vi "GEA3 HEWH Standard ERDs.vi"(8 "Error In":errorcluster, 10 "ERD Data Input":T1[](array[typedef]) {"ERD Number" format="%.0x"}, 11 "ERD Data  in":T2) -> (0 "Error Out":errorcluster, 2 "ERD Data Output":T1[](array[typedef]) {"ERD Number" format="%.0x"}, 3 "ERD Data  out":T2, 5 "Standard Data":string[][](array[string]))   [LabVIEW 2020]
uses:
  type defs/ERD Read Data Out.ctl
  Type Definitions/GEA3 HEWH ERD Data.ctl
  Type Definitions/GEA3 HEWH Mixing Valve.ctl
  library/GEA2_Toolkit.lvlib
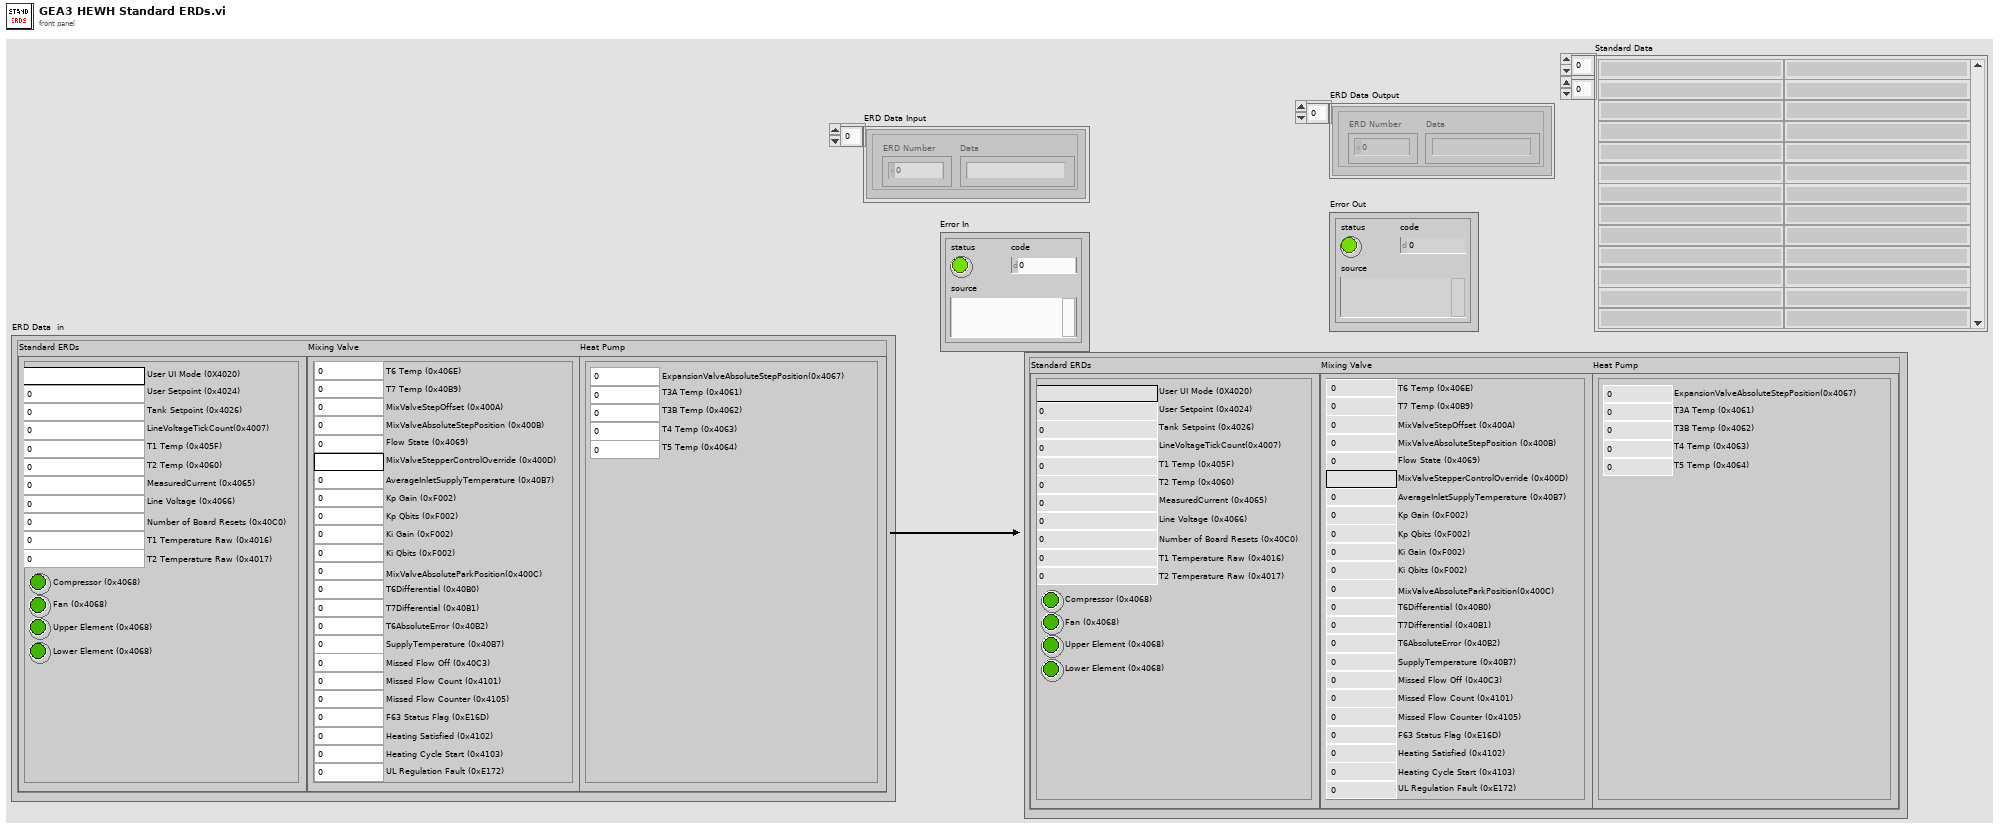
[diagram p1: front panel]
types:
  T1 = typedef "GEA2_Toolkit.lvlib/ERD Read Data Out.ctl" = cluster{"ERD Number":u16, "Data":string}
  T2 = typedef "GEA3 HEWH ERD Data.ctl" = cluster{"Mixing Valve":T3, "Standard ERDs":cluster{"User UI Mode (0X4020)":string, "User Setpoint (0x4024)":u16, "Compressor (0x4068)":bool, "Lower Element (0x4068)":bool, "Upper Element (0x4068)":bool, "Fan (0x4068)":bool, "T1 Temp (0x405F)":dbl, "T2 Temp (0x4060)":dbl, "Line Voltage (0x4066)":dbl, "MeasuredCurrent (0x4065)":dbl, "LineVoltageTickCount(0x4007)":u16, "Number of Board Resets (0x40C0)":u16, "T1 Temperature Raw (0x4016)":u16, "T2 Temperature Raw (0x4017)":u16, "Tank Setpoint (0x4026)":u16}, "Heat Pump":cluster{"ExpansionValveAbsoluteStepPosition(0x4067)":i16, "T3A Temp (0x4061)":dbl, "T3B Temp (0x4062)":dbl, "T4 Temp (0x4063)":dbl, "T5 Temp (0x4064)":dbl}}
  T3 = typedef "GEA3 HEWH Mixing Valve.ctl" = cluster{"T7 Temp (0x40B9)":dbl, "MixValveStepOffset (0x400A)":i16, "MixValveAbsoluteStepPosition (0x400B)":i16, "Flow State (0x4069)":u8, "MixValveStepperControlOverride (0x400D)":string, "AverageInletSupplyTemperature (0x40B7)":dbl, "T6 Temp (0x406E)":dbl, "Kp Gain (0xF002)":u16, "Kp Qbits (0xF002)":u16, "Ki Gain (0xF002)":u16, "Ki Qbits (0xF002)":u16, "MixValveAbsoluteParkPosition(0x400C)":i16, "T7Differential (0x40B1)":dbl, "T6Differential (0x40B0)":dbl, "SupplyTemperature (0x40B7)":dbl, "Missed Flow Off (0x40C3)":u8, "T6AbsoluteError (0x40B2)":dbl, "Missed Flow Count (0x4101)":u16, "Missed Flow Counter (0x4105)":u16, "F63 Status Flag (0xE16D)":u16, "Heating Satisfied (0x4102)":u16, "Heating Cycle Start (0x4103)":u16, "UL Regulation Fault (0xE172)":u8}
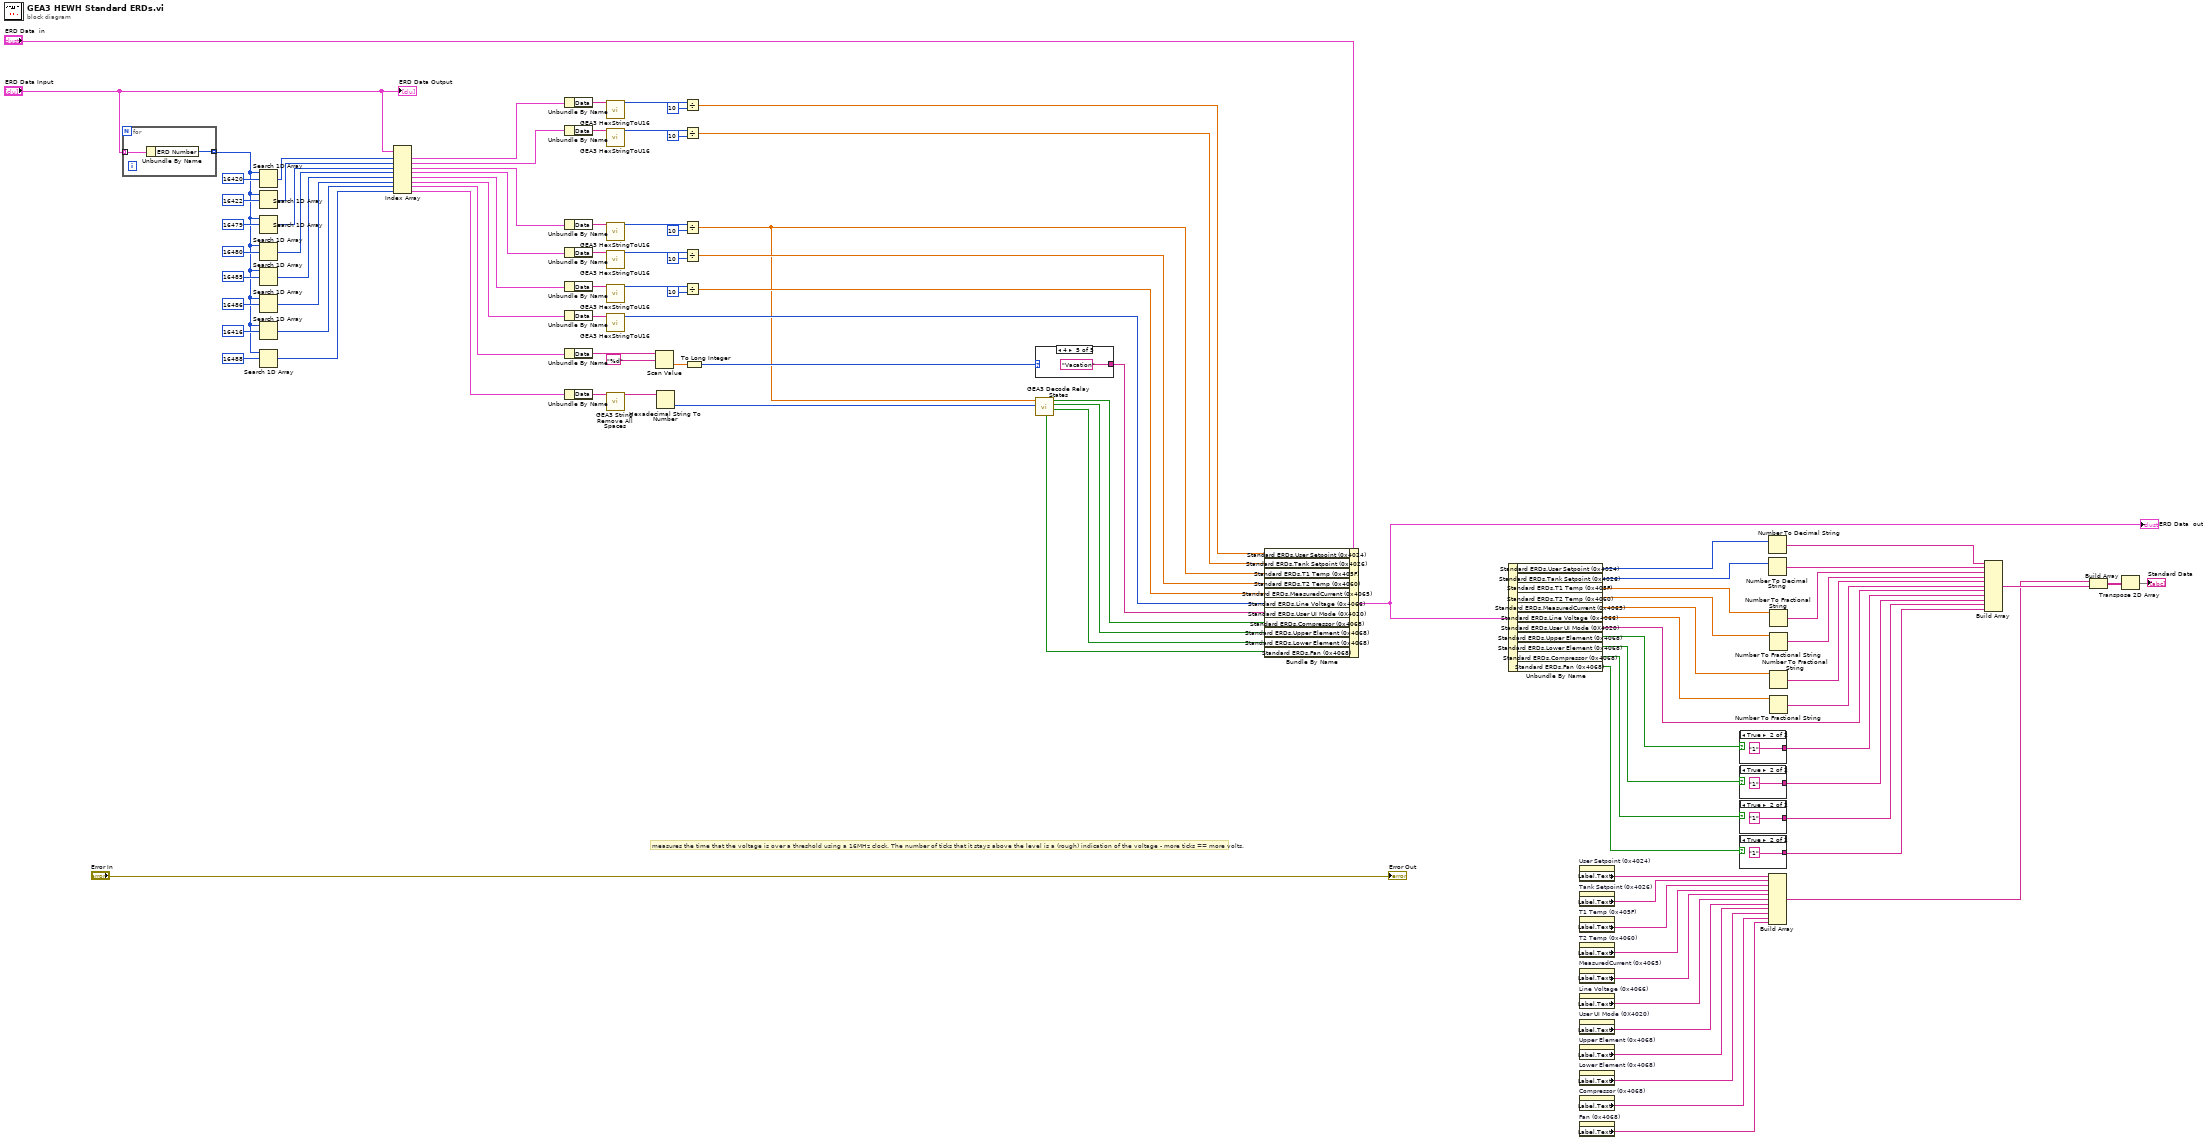
[diagram p0: block diagram]
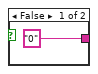
[diagram p2: hidden frame]
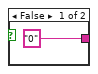
[diagram p3: hidden frame]
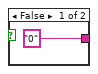
[diagram p4: hidden frame]
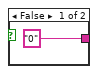
[diagram p5: hidden frame]
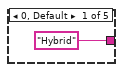
[diagram p6: hidden frame]
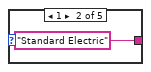
[diagram p7: hidden frame]
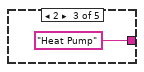
[diagram p8: hidden frame]
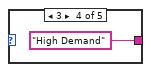
[diagram p9: hidden frame]
diagram:
  # "measures the time that the voltage is over a threshold using a 16MHz clock. The number of ticks that it stays above the level is a (rough) indication of the voltage - more ticks == more volts."
  n1 = for {
    tunnel: "ERD Data Input" -> [w101] mode=indexing
    tunnel: [w100] -> w23 mode=indexing
    n2 = Unbundle By Name(w101) -> ("ERD Number"=w100:u16)
  }
  n3 = Search 1D Array(1D array=w23, element=u16 16420 ("ERD Number")) -> (index of element=w43:i32)  [unwired: 1 in]
  n4 = Search 1D Array(1D array=w23, element=u16 16422 ("ERD Number")) -> (index of element=w31:i32)  [unwired: 1 in]
  n5 = Search 1D Array(1D array=w23, element=u16 16479 ("ERD Number")) -> (index of element=w22:i32)  [unwired: 1 in]
  n6 = Search 1D Array(1D array=w23, element=u16 16480 ("ERD Number")) -> (index of element=w21:i32)  [unwired: 1 in]
  n7 = Search 1D Array(1D array=w23, element=u16 16485 ("ERD Number")) -> (index of element=w20:i32)  [unwired: 1 in]
  n8 = Search 1D Array(1D array=w23, element=u16 16486 ("ERD Number")) -> (index of element=w19:i32)  [unwired: 1 in]
  n9 = Search 1D Array(1D array=w23, element=u16 16416 ("ERD Number")) -> (index of element=w18:i32)  [unwired: 1 in]
  n10 = Search 1D Array(1D array=w23, element=u16 16488 ("ERD Number")) -> (index of element=w17:i32)  [unwired: 1 in]
  n11 = Index Array(array="ERD Data Input", index #1=w43, index #2=w31, index #3=w22, index #4=w21, index #5=w20, index #6=w19, index #7=w18, index #8=w17) -> (element #1=w42:T1, element #2=w27:T1, element #3=w16:T1, element #4=w15:T1, element #5=w14:T1, element #6=w13:T1, element #7=w12:T1, element #8=w11:T1)
  n12 = Unbundle By Name(w42) -> ("Data"=w79:string)
  n13 = Unbundle By Name(w27) -> ("Data"=w28:string)
  n14 = Unbundle By Name(w16) -> ("Data"=w75:string)
  n15 = Unbundle By Name(w15) -> ("Data"=w81:string)
  n16 = Unbundle By Name(w14) -> ("Data"=w86:string)
  n17 = Unbundle By Name(w13) -> ("Data"=w88:string)
  n18 = Unbundle By Name(w12) -> ("Data"=w90:string)
  n19 = Unbundle By Name(w11) -> ("Data"=w94:string)
  n20 = call "GEA3 HexStringToU16.vi"("Input String"=w79) -> ("Number Out"=w77:u16)  [unwired: 14 in]
  n21 = call "GEA3 HexStringToU16.vi"("Input String"=w28) -> ("Number Out"=w30:u16)  [unwired: 14 in]
  n22 = call "GEA3 HexStringToU16.vi"("Input String"=w75) -> ("Number Out"=w73:u16)  [unwired: 14 in]
  n23 = call "GEA3 HexStringToU16.vi"("Input String"=w81) -> ("Number Out"=w83:u16)  [unwired: 14 in]
  n24 = call "GEA3 HexStringToU16.vi"("Input String"=w86) -> ("Number Out"=w85:u16)  [unwired: 14 in]
  n25 = call "GEA3 HexStringToU16.vi"("Input String"=w88) -> ("Number Out"=w89:u16)  [unwired: 14 in]
  n26 = call "GEA3 String Remove All Spaces.vi"("Input String"=w94) -> ("Spaces Removed"=w93:string)  [unwired: 13 in, 1 out]
  n27 = Scan Value(string=w90, format string="%d") -> (value=w95:dbl)  [unwired: 1 in, 1 out]
  n28 = Hexadecimal String To Number(string=w93) -> (number=w92:u32)  [unwired: 2 in, 1 out]
  n29 = Divide(x=w77, y=u16 10) -> (x/y=w80:dbl)
  n30 = Divide(x=w30, y=u16 10) -> (x/y=w26:dbl)
  n31 = Divide(x=w73, y=u16 10) -> (x/y=w64:dbl)
  n32 = Divide(x=w83, y=u16 10) -> (x/y=w76:dbl)
  n33 = Divide(x=w85, y=u16 10) -> (x/y=w87:dbl)
  n34 = To Long Integer(number=w95) -> (32bit integer=w96:i32)
  n35 = case shown="4" w96 {
    tunnel: ["Hybrid" "Standard Electric" "Heat Pump" "High Demand" "Vacation"] -> w97
    frame 0, Default {
    }
    frame 1 {
    }
    frame 2 {
    }
    frame 3 {
    }
    frame 4 {
    }
  }
  n36 = call "GEA3 Decode Relay States.vi"("ERD Relay Value"=w92, "T1 Temp"=w64) -> ("Lower Element (0x4033)"=w39:bool, "Upper Element (0x4033)"=w38:bool, "Compressor (0x4033)"=w40:bool, "Fan (0x4033)"=w37:bool)  [unwired: 6 in]
  n37 = Bundle By Name(cluster="ERD Data  in", "Standard ERDs.User Setpoint (0x4024)"=w80, "Standard ERDs.Tank Setpoint (0x4026)"=w26, "Standard ERDs.T1 Temp (0x405F)"=w64, "Standard ERDs.T2 Temp (0x4060)"=w76, "Standard ERDs.MeasuredCurrent (0x4065)"=w87, "Standard ERDs.Line Voltage (0x4066)"=w89, "Standard ERDs.User UI Mode (0X4020)"=w97, "Standard ERDs.Compressor (0x4068)"=w40, "Standard ERDs.Upper Element (0x4068)"=w38, "Standard ERDs.Lower Element (0x4068)"=w39, "Standard ERDs.Fan (0x4068)"=w37) -> (w63:T2)
  "ERD Data  out" <- w63
  n38 = Unbundle By Name(w63) -> ("Standard ERDs.User Setpoint (0x4024)"=w62:u16, "Standard ERDs.Tank Setpoint (0x4026)"=w25:u16, "Standard ERDs.T1 Temp (0x405F)"=w61:dbl, "Standard ERDs.T2 Temp (0x4060)"=w60:dbl, "Standard ERDs.MeasuredCurrent (0x4065)"=w59:dbl, "Standard ERDs.Line Voltage (0x4066)"=w58:dbl, "Standard ERDs.User UI Mode (0X4020)"=w52:string, "Standard ERDs.Upper Element (0x4068)"=w51:bool, "Standard ERDs.Lower Element (0x4068)"=w49:bool, "Standard ERDs.Compressor (0x4068)"=w36:bool, "Standard ERDs.Fan (0x4068)"=w35:bool)
  n39 = property on="User Setpoint (0x4024)" class="DigNum (strict)"() -> ("Label.Text"=w41:string)  [unwired: 2 in, 2 out]
  n40 = property on="Tank Setpoint (0x4026)" class="DigNum (strict)"() -> ("Label.Text"=w10:string)  [unwired: 2 in, 2 out]
  n41 = property on="T1 Temp (0x405F)" class="DigNum (strict)"() -> ("Label.Text"=w9:string)  [unwired: 2 in, 2 out]
  n42 = property on="T2 Temp (0x4060)" class="DigNum (strict)"() -> ("Label.Text"=w8:string)  [unwired: 2 in, 2 out]
  n43 = property on="MeasuredCurrent (0x4065)" class="DigNum (strict)"() -> ("Label.Text"=w7:string)  [unwired: 2 in, 2 out]
  n44 = property on="Line Voltage (0x4066)" class="DigNum (strict)"() -> ("Label.Text"=w6:string)  [unwired: 2 in, 2 out]
  n45 = property on="User UI Mode (0X4020)" class="Str"() -> ("Label.Text"=w5:string)  [unwired: 2 in, 2 out]
  n46 = property on="Upper Element (0x4068)" class="Bool (strict)"() -> ("Label.Text"=w4:string)  [unwired: 2 in, 2 out]
  n47 = property on="Lower Element (0x4068)" class="Bool (strict)"() -> ("Label.Text"=w3:string)  [unwired: 2 in, 2 out]
  n48 = property on="Compressor (0x4068)" class="Bool (strict)"() -> ("Label.Text"=w2:string)  [unwired: 2 in, 2 out]
  n49 = property on="Fan (0x4068)" class="Bool (strict)"() -> ("Label.Text"=w1:string)  [unwired: 2 in, 2 out]
  n50 = case shown="True" w51 {
    tunnel: ["0" "1"] -> w50
    frame False {
    }
    frame True {
    }
  }
  n51 = case shown="True" w49 {
    tunnel: ["0" "1"] -> w48
    frame False {
    }
    frame True {
    }
  }
  n52 = case shown="True" w36 {
    tunnel: ["0" "1"] -> w34
    frame False {
    }
    frame True {
    }
  }
  n53 = case shown="True" w35 {
    tunnel: ["0" "1"] -> w33
    frame False {
    }
    frame True {
    }
  }
  n54 = Number To Decimal String(number=w62) -> (decimal integer string=w57:string)  [unwired: 1 in]
  n55 = Number To Decimal String(number=w25) -> (decimal integer string=w24:string)  [unwired: 1 in]
  n56 = Build Array(w41, w10, w9, w8, w7, w6, w5, w4, w3, w2, w1) -> (w46:string[])
  n57 = Number To Fractional String(number=w61) -> (F-format string=w56:string)  [unwired: 3 in]
  n58 = Number To Fractional String(number=w60) -> (F-format string=w55:string)  [unwired: 3 in]
  n59 = Number To Fractional String(number=w59) -> (F-format string=w54:string)  [unwired: 3 in]
  n60 = Number To Fractional String(number=w58) -> (F-format string=w53:string)  [unwired: 3 in]
  n61 = Build Array(w57, w24, w56, w55, w54, w53, w52, w50, w48, w34, w33) -> (w47:string[])
  n62 = Build Array(w46, w47) -> (w45:string[][])
  n63 = Transpose 2D Array(2D array=w45) -> (transposed array=→"Standard Data":string[][])
  "Error Out" <- "Error In"
  "ERD Data Output" <- "ERD Data Input"
